vi "z_stack_ OG_waveform_old.vi"(0 "Bi-lateral Z galvo scan volt":dbl, 1 "Objective 线性减速 时间（s）":dbl, 2 "Steps per Volume":dbl, 3 "OG Z stack 线性加速 采样信息":cluster{"采样率":dbl, "采样数":dbl}, 4 "OG Z stack 刺激steps 采样信息":cluster{"采样率":dbl, "采样数":dbl}, 6 "OG Z stack 线性减速 采样信息":cluster{"采样率":dbl, "采样数":dbl}, 7 "OG start layer":dbl, 9 "Objective volet 线性减速 时间（s）":dbl, 10 "OG end layer":dbl, 11 "OG repitation":dbl, 12 "Objective 刺激steps 时间（s）":dbl, 13 "Objective 线性加速 时间（s）":dbl) -> (14 "waveform out":waveform(dbl))   [LabVIEW 2012]
uses:
  <vilib>/Waveform/WDTOps.llb/WDT Append Waveforms DBL.vi
  <vilib>/measure/NI_MABase.lvlib
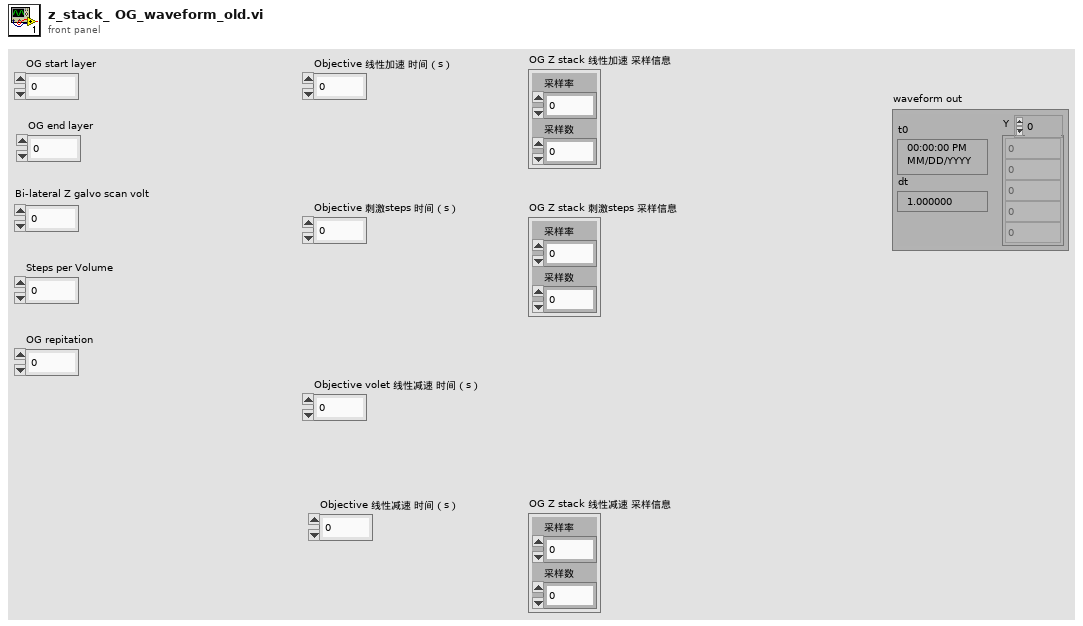
[diagram p1: front panel]
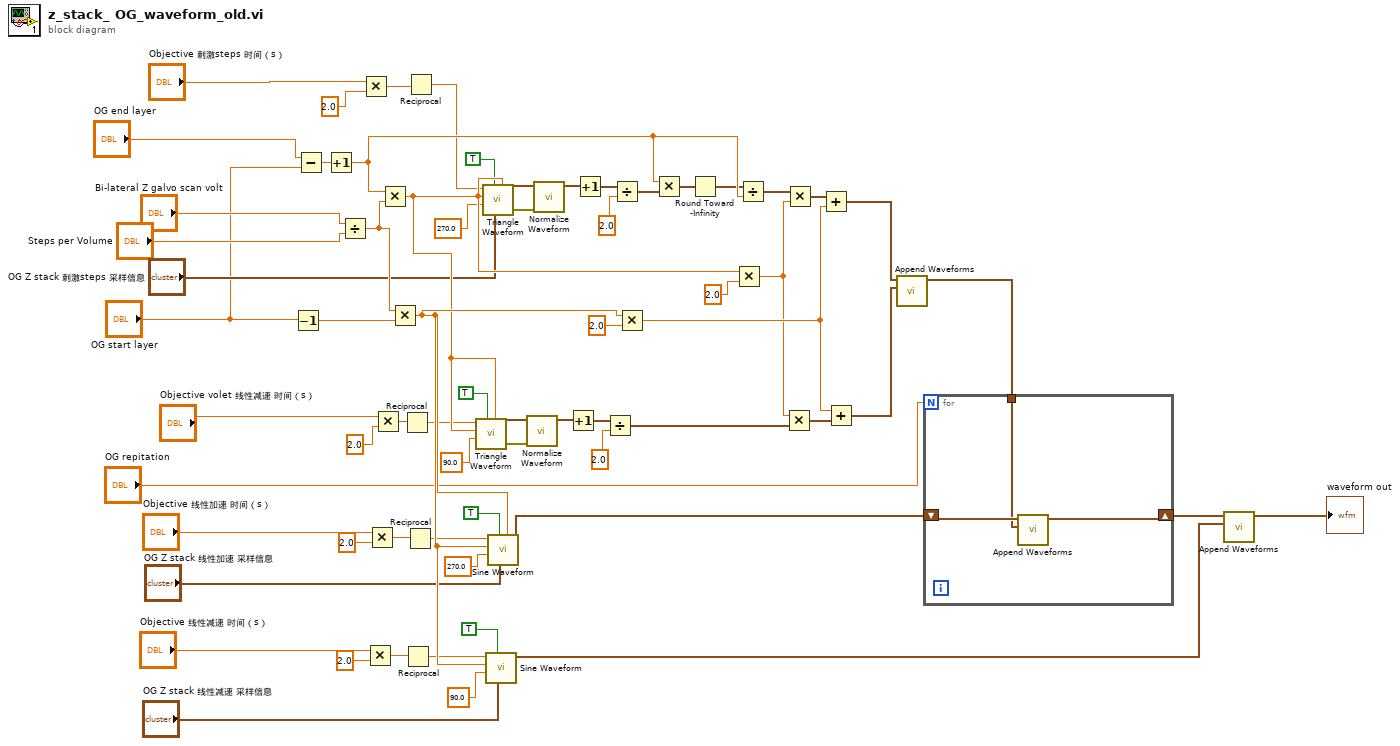
[diagram p0: block diagram]
diagram:
  n1 = Decrement(x="OG start layer") -> (x-1=w26:dbl)
  n2 = Subtract(x="OG end layer", y="OG start layer") -> (x-y=w22:dbl)
  n3 = Increment(x=w22) -> (x+1=w24:dbl)
  n4 = Divide(x="Bi-lateral Z galvo scan volt", y="Steps per Volume") -> (x/y=w25:dbl)
  n5 = Multiply(x="Objective 刺激steps 时间（s）", y=2.0 ("phase")) -> (x*y=w16:dbl)
  n6 = Multiply(x="Objective 线性减速 时间（s）", y=2.0) -> (x*y=w35:dbl)
  n7 = Multiply(x="Objective 线性加速 时间（s）", y=2.0) -> (x*y=w30:dbl)
  n8 = Multiply(x="Objective volet 线性减速 时间（s）", y=2.0) -> (x*y=w46:dbl)
  n9 = Multiply(x=w24, y=w25) -> (x*y=w48:dbl)
  n10 = Multiply(x=w25, y=w26) -> (x*y=w61:dbl)
  n11 = Reciprocal(x=w46) -> (1/x=w47:dbl)
  n12 = Reciprocal(x=w35) -> (1/x=w36:dbl)
  n13 = Reciprocal(x=w30) -> (1/x=w31:dbl)
  n14 = Reciprocal(x=w16) -> (1/x=w15:dbl)
  n15 = call <vilib>:"Triangle Waveform.vi"("offset"=w48, "reset signal"=TRUE, "phase"=90.0, "amplitude"=w48, "frequency"=w47) -> ("error out"=w40:errorcluster, "signal out"=w41:waveform(dbl))  [unwired: 5 in]
  n16 = call <vilib>:"Triangle Waveform.vi"("offset"=w48, "sampling info"="OG Z stack 刺激steps 采样信息", "reset signal"=TRUE, "phase"=270.0, "amplitude"=w48, "frequency"=w15) -> ("error out"=w11:errorcluster, "signal out"=w12:waveform(dbl))  [unwired: 4 in]
  n17 = call <vilib>:"Sine Waveform.vi"("sampling info"="OG Z stack 线性减速 采样信息", "reset signal"=TRUE, "phase"=90.0, "amplitude"=w61, "frequency"=w36) -> ("signal out"=w63:waveform(dbl))  [unwired: 5 in, 1 out]
  n18 = call <vilib>:"Sine Waveform.vi"("offset"=w61, "sampling info"="OG Z stack 线性加速 采样信息", "reset signal"=TRUE, "phase"=270.0, "amplitude"=w61, "frequency"=w31) -> ("signal out"=w60:waveform(dbl))  [unwired: 4 in, 1 out]
  n19 = call <vilib>:"Normalize Waveform.vi"("error in (no error)"=w40, "waveform in"=w41) -> ("normalized waveform"=w39:waveform(dbl))  [unwired: 6 in, 3 out]
  n20 = call <vilib>:"Normalize Waveform.vi"("error in (no error)"=w11, "waveform in"=w12) -> ("normalized waveform"=w10:waveform(dbl))  [unwired: 6 in, 3 out]
  n21 = Increment(x=w39) -> (x+1=w38:waveform(dbl))
  n22 = Increment(x=w10) -> (x+1=w9:waveform(dbl))
  n23 = Divide(x=w38, y=2.0 ("phase")) -> (x/y=w49:waveform(dbl))
  n24 = Divide(x=w9, y=2.0 ("phase")) -> (x/y=w8:waveform(dbl))
  n25 = Multiply(x=w61, y=2.0) -> (x*y=w52:dbl)
  n26 = Multiply(x=w24, y=w8) -> (x*y=w7:waveform(dbl))
  n27 = Round Toward -Infinity(1:w7) -> (0:w6:waveform(dbl))
  n28 = Multiply(x=w48, y=2.0 ("phase")) -> (x*y=w50:dbl)
  n29 = Divide(x=w6, y=w24) -> (x/y=w4:waveform(dbl))
  n30 = Multiply(x=w50, y=w49) -> (x*y=w51:waveform(dbl))
  n31 = Multiply(x=w4, y=w50) -> (x*y=w5:waveform(dbl))
  n32 = Add(x=w5, y=w52) -> (x+y=w53:waveform(dbl))
  n33 = Add(x=w52, y=w51) -> (x+y=w54:waveform(dbl))
  n34 = call-poly <vilib>:"Append Waveforms.vi"("waveform B"=w54, "waveform A"=w53) -> ("waveform out"=w55:waveform(dbl))  [unwired: 8 in, 1 out]
  n35 = for {
    N: "OG repitation" -> [_]
    tunnel: w55 -> [w68]
    shift-right: [w67] -> w56
    shift-left: w60 -> [w69]
    n36 = call-poly <vilib>:"Append Waveforms.vi"("waveform B"=w68, "waveform A"=w69) -> ("waveform out"=w67:waveform(dbl))  [unwired: 8 in, 1 out]
  }
  n37 = call-poly <vilib>:"Append Waveforms.vi"("waveform B"=w63, "waveform A"=w56) -> ("waveform out"=→"waveform out":waveform(dbl))  [unwired: 8 in, 1 out]
